vi "Client - Main.vi"(8 "error in (no error)":errorcluster) -> (0 "error out":errorcluster)   [LabVIEW 2019]
doc: "This VI should be run on the client PC."
panel:
  out "log file path":path
  out "log file name":string
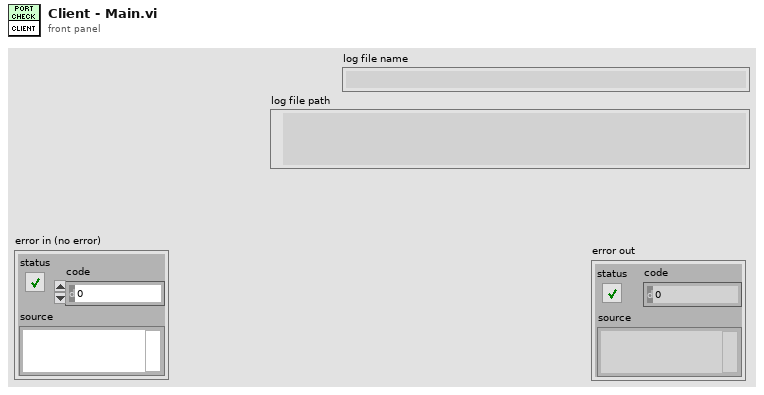
[diagram p1: front panel]
types:
  T1 = typedef "Ports to Check.ctl" = cluster{"TCP Ports":u32[], "UDP Ports":u32[]}
  T2 = typedef "Results.ctl" = T3[]
  T3 = typedef "log data cluster.ctl" = cluster{"Time Stamp":timestamp, "Port Number":u16, "Communication Type":T4, "success?":bool, "error in":errorcluster}
  T4 = typedef "Communication Types.ctl" = enum16{"UDP - Server to Client", "UDP - Client to Server", "TCP - Server to Client", "TCP - Client to Server"}
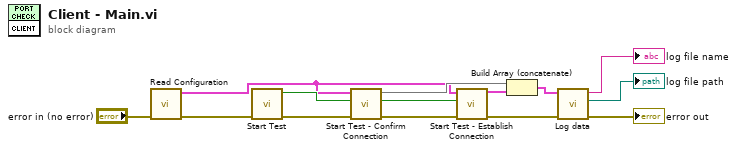
[diagram p0: block diagram]
diagram:
  n1 = call "Read Configuration.vi"("error in (no error)"="error in (no error)") -> ("error out"=w14:errorcluster, "Ports to Check"=w6:T1)  [unwired: 9 in]
  n2 = call "Start Test.vi"("error in (no error)"=w14) -> ("error out"=w13:errorcluster, "Connection Established?"=w12:bool)  [unwired: 9 in]
  n3 = call "Start Test - Confirm Connection.vi"(0:w6, 1:w12, "error in (no error)"=w13) -> (7:w11, "Connection Established"=w7:bool, "error out"=w9:errorcluster)  [unwired: 4 in, 1 out]
  n4 = call "Start Test - Establish Connection.vi"("Ports to Check"=w6, "Connection Established?"=w7, "error in (no error)"=w9) -> ("Results"=w1:T2, "error out"=w8:errorcluster)  [unwired: 5 in, 1 out]
  n5 = Build Array (concatenate)(w11, w1) -> (w10:T2)
  n6 = call "Log data.vi"("error in (no error)"=w8, "Results"=w10) -> ("error out"=→"error out":errorcluster, "log file path"=→"log file path":path, "log file name"=→"log file name":string)  [unwired: 7 in]
